vi "Output Enable Read Single.vi"(8 "error in":errorcluster, 9 "Channel Index":i32=1, 11 "Cycler in":refnum<class "Cycler.lvclass">) -> (0 "error out":errorcluster, 1 "Changed or First Call?":bool, 2 "Output Enable ACT":bool, 3 "Cycler out":refnum<class "Cycler.lvclass">)   [LabVIEW 2023, in "Cycler.lvclass"]
uses:
  Cycler.lvclass
  Low Level Capabilities/Output Enable/Output Enable.lvclass
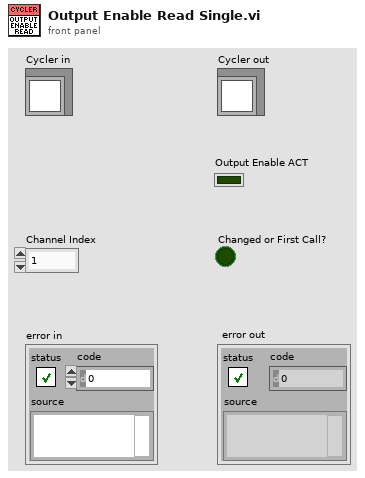
[diagram p1: front panel]
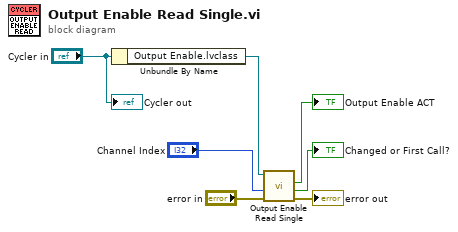
[diagram p0: block diagram]
diagram:
  n1 = Unbundle By Name("Cycler in") -> ("Output Enable.lvclass"=w2:refnum<class "Output Enable.lvclass">)
  n2 = call-dynamic "Output Enable Read Single.vi"("error in"="error in", "Channel Index"="Channel Index", "Output Enable in"=w2) -> ("error out"=→"error out":errorcluster, "Changed or First Call?"=→"Changed or First Call?":bool, "Output Enable ACT"=→"Output Enable ACT":bool)  [unwired: 5 in, 1 out]
  "Cycler out" <- "Cycler in"
